vi "USBCom.vi"(0 "VISA resource name":refnum<visa-resource-name>, 5 "command":string, 11 "error in (no error)":errorcluster) -> (15 "error out":errorcluster)   [LabVIEW 2018]
uses:
  <vilib>/Instr/_visa.llb/VISA Flush IO Buffer Mask.ctl
  <vilib>/Instr/_visa.llb/VISA Configure Serial Port (Instr).vi
panel:
  in  "Add 0D0A":bool
  out "write buffer":string
  out "binary[7]":string
  out "number[7]":u32
  out "byte[7]":string
  out "number[4]":u32
  out "number[5]":u32
  out "number[6]":u32
  out "binary[6]":string
  out "byte[6]":string
  out "binary[5]":string
  out "byte[5]":string
  out "byte[4]":string
  out "binary[4]":string
  in  "resetValues":bool
  out "binary[3]":string
  out "number[3]":u32
  out "byte[3]":string
  out "number[0]":u32
  out "number[1]":u32
  out "number[2]":u32
  out "binary[2]":string
  out "byte[2]":string
  out "binary[1]":string
  out "byte[1]":string
  out "byte[0]":string
  out "binary[0]":string
  out "byte Array":string[](array[string])
  out "valid byte":string
  out "bytes at port":u32
  out "byte count":u32
  out "read buffer":string
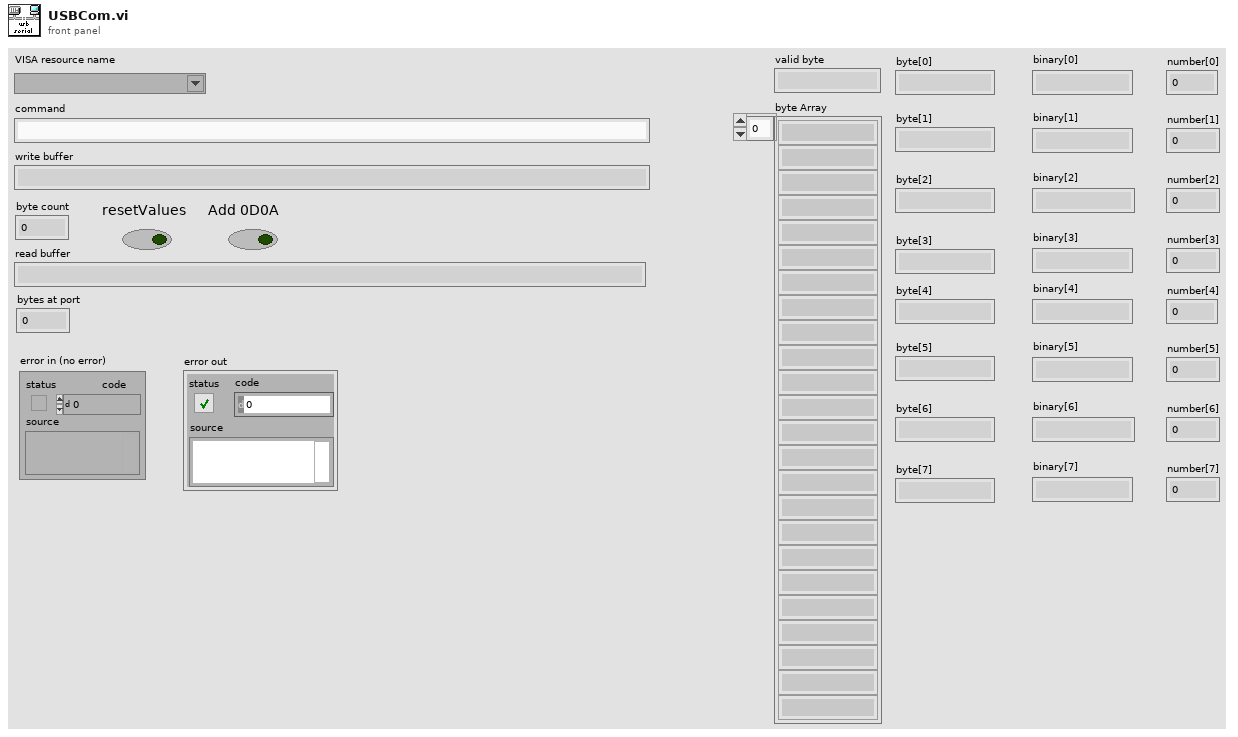
[diagram p1: front panel]
types:
  T1 = typedef "VISA Flush IO Buffer Mask.ctl" = u16
  T2 = cluster{"[0]":string, "[1]":string, "[2]":string, "[3]":string, "[4]":string, "[5]":string, "[6]":string, "[7]":string, "[8]":string}
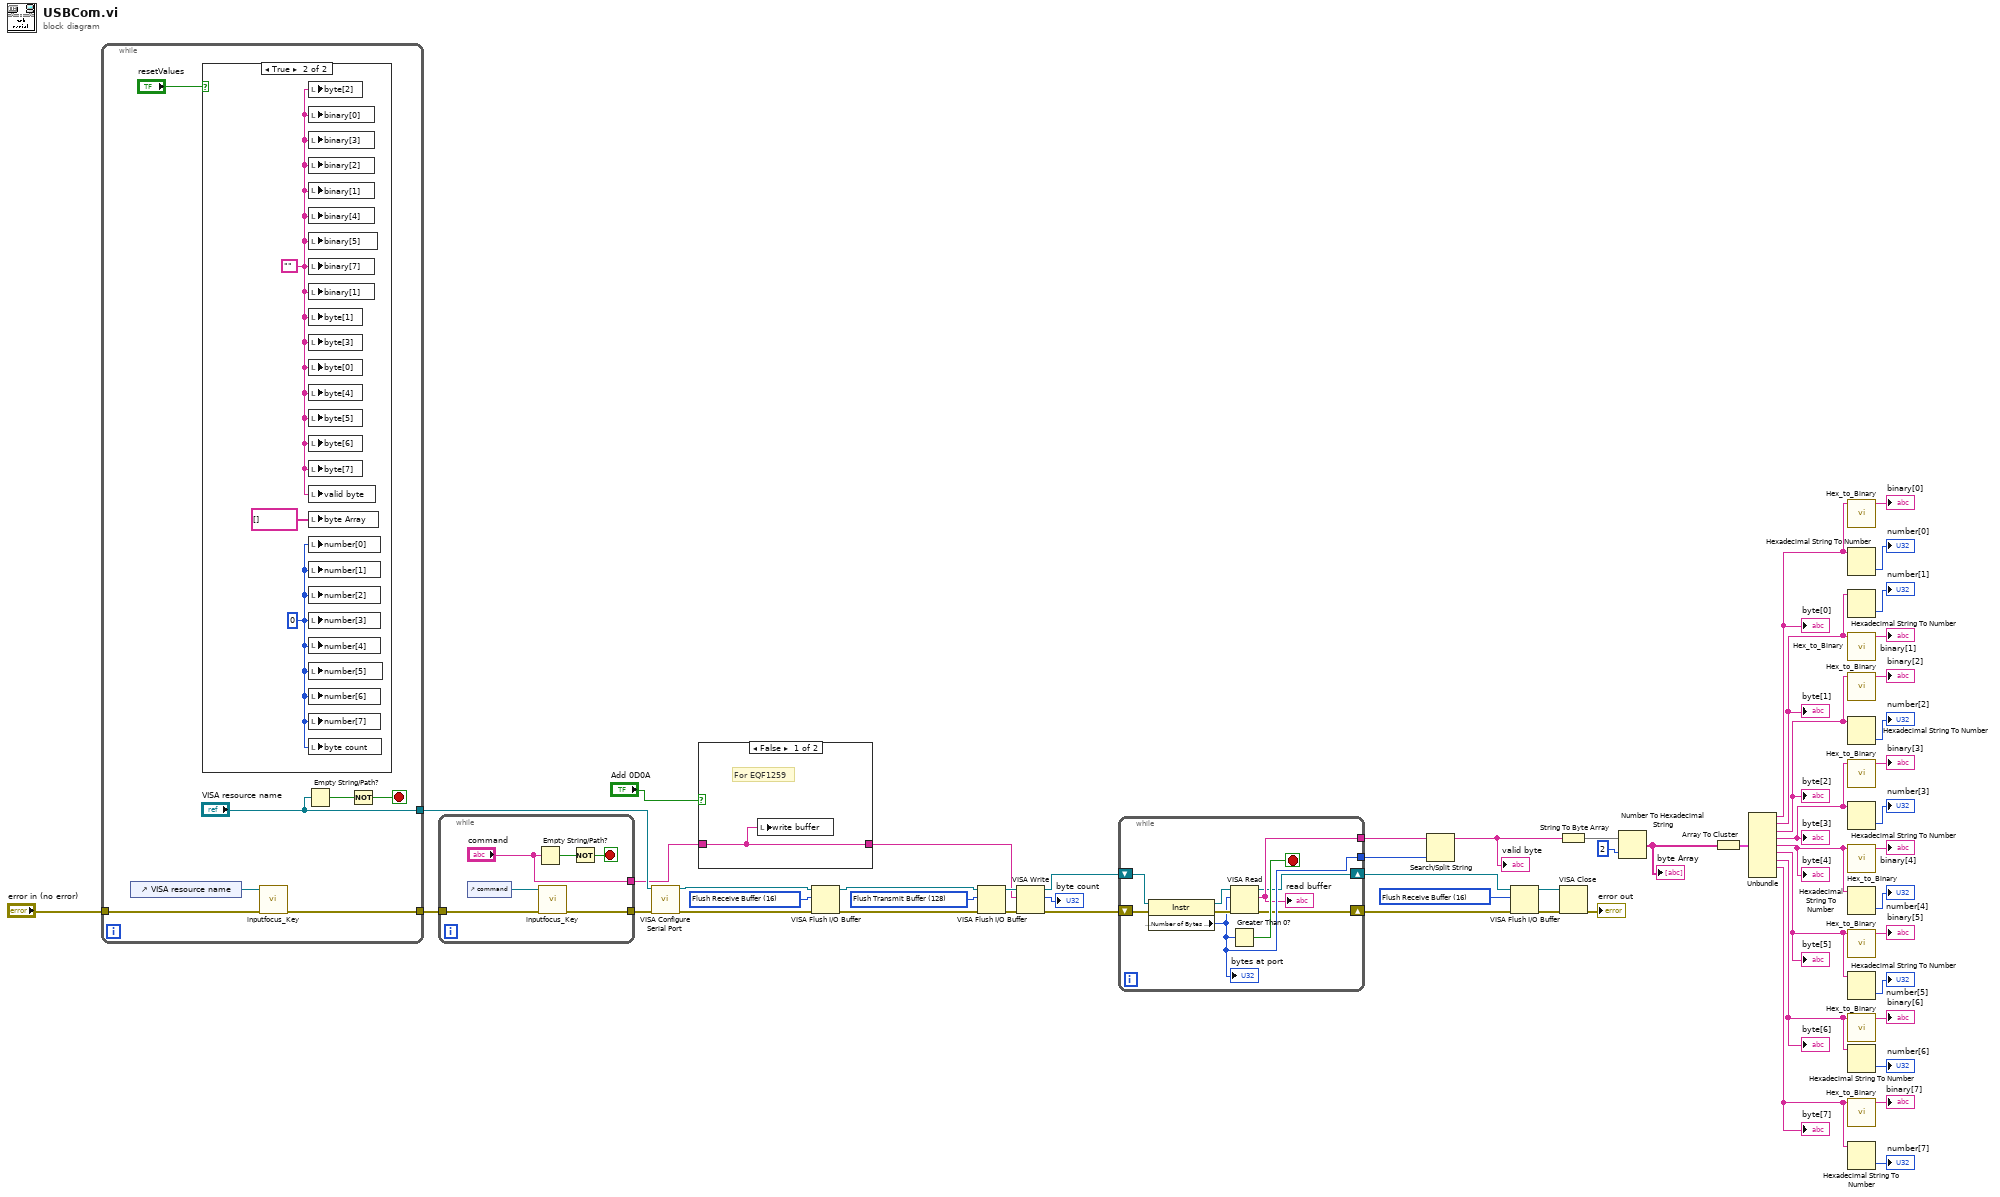
[diagram p0: block diagram]
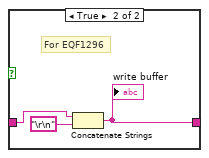
[diagram p2: hidden frame]
diagram:
  w39 = T1 128 items=["Flush Receive Buffer"=16, "Write Transmit Buffer to Device"=32, "Flush Receive Buffer (No I/O)"=64, "Flush Transmit Buffer"=128] ("Mask")
  w43 = T1 16 items=["Flush Receive Buffer"=16, "Write Transmit Buffer to Device"=32, "Flush Receive Buffer (No I/O)"=64, "Flush Transmit Buffer"=128] ("Mask")
  w46 = T1 16 items=["Flush Receive Buffer"=16, "Write Transmit Buffer to Device"=32, "Flush Receive Buffer (No I/O)"=64, "Flush Transmit Buffer"=128] ("Mask")
  n1 = while {
    tunnel: ["VISA resource name"] -> w33
    tunnel: [w62] -> w32
    tunnel: "error in (no error)" -> [w61]
    stop <- w57 stop-if-true
    n2 = control-ref of="VISA resource name"() -> (w60:refnum<vi>)
    n3 = case shown="True" "resetValues" {
      frame False {
      }
      frame True {
        w64 = u32 0
        w63 = ""
        n4 = local write "byte[2]"(w63) -> ()
        n5 = local write "binary[0]"(w63) -> ()
        n6 = local write "binary[3]"(w63) -> ()
        n7 = local write "binary[2]"(w63) -> ()
        n8 = local write "binary[1]"(w63) -> ()
        n9 = local write "binary[4]"(w63) -> ()
        n10 = local write "binary[5]"(w63) -> ()
        n11 = local write "binary[7]"(w63) -> ()
        n12 = local write "binary[1]"(w63) -> ()
        n13 = local write "byte[1]"(w63) -> ()
        n14 = local write "byte[3]"(w63) -> ()
        n15 = local write "byte[0]"(w63) -> ()
        n16 = local write "byte[4]"(w63) -> ()
        n17 = local write "byte[5]"(w63) -> ()
        n18 = local write "byte[6]"(w63) -> ()
        n19 = local write "byte[7]"(w63) -> ()
        n20 = local write "valid byte"(w63) -> ()
        n21 = local write "byte Array"(string[] []) -> ()
        n22 = local write "number[0]"(w64) -> ()
        n23 = local write "number[1]"(w64) -> ()
        n24 = local write "number[2]"(w64) -> ()
        n25 = local write "number[3]"(w64) -> ()
        n26 = local write "number[4]"(w64) -> ()
        n27 = local write "number[5]"(w64) -> ()
        n28 = local write "number[6]"(w64) -> ()
        n29 = local write "number[7]"(w64) -> ()
        n30 = local write "byte count"(w64) -> ()
      }
    }
    n31 = call "inputfocus_Key.vi"("error in (no error)"=w61, "reference"=w60) -> ("error out"=w62:errorcluster)  [unwired: 9 in]
    n32 = Empty String/Path?(string/path="VISA resource name") -> (empty?=w58:bool)
    n33 = Not(x=w58) -> (.not. x?=w57:bool)
  }
  n34 = while {
    tunnel: ["command"] -> w3
    tunnel: w32 -> [w71]
    tunnel: [w70] -> w31
    stop <- w66 stop-if-true
    n35 = control-ref of="command"() -> (w69:refnum<vi>)
    n36 = Empty String/Path?(string/path="command") -> (empty?=w67:bool)
    n37 = call "inputfocus_Key.vi"("error in (no error)"=w71, "reference"=w69) -> ("error out"=w70:errorcluster)  [unwired: 9 in]
    n38 = Not(x=w67) -> (.not. x?=w66:bool)
  }
  n39 = call-poly "VISA Configure Serial Port"("VISA resource name"=w33, "error in (no error)"=w31) -> ("VISA resource name out"=w45:refnum<visa-resource-name>, "error out"=w44:errorcluster)  [unwired: 12 in]
  n40 = case shown="False" "Add 0D0A" {
    tunnel: w3 -> [w72 w74]
    tunnel: [w72 w73] -> w2
    frame False {
      # "For EQF1259"
      n41 = local write "write buffer"(w72) -> ()
    }
    frame True {
      # "For EQF1296"
      n42 = Concatenate Strings(w74, "\r\n") -> (w73:string)
      "write buffer" <- w73
    }
  }
  n43 = VISA Flush I/O Buffer(VISA resource name=w45, mask (16)=w43, error in (no error)=w44) -> (VISA resource name out=w40:refnum<visa-resource-name>, error out=w41:errorcluster)
  n44 = VISA Flush I/O Buffer(VISA resource name=w40, mask (16)=w39, error in (no error)=w41) -> (VISA resource name out=w38:refnum<visa-resource-name>, error out=w37:errorcluster)
  n45 = VISA Write(VISA resource name=w38, write buffer=w2, error in (no error)=w37) -> (VISA resource name out=w55:refnum<visa-resource-name>, return count=→"byte count":u32, error out=w54:errorcluster)
  n46 = while {
    tunnel: [w78] -> w4
    tunnel: [w79] -> w50
    shift-right: [w76] -> w42
    shift-left: w55 -> [w84]
    shift-right: [w77] -> w47
    shift-left: w54 -> [w83]
    stop <- w80 stop-if-true
    n47 = property class="Instr"(reference=w84, error in=w83) -> (reference out=w81:refnum<visa-resource-name>, error out=w82:errorcluster, "Serial Settings:Number of Bytes at Serial Port"=w79:u32)
    "bytes at port" <- w79
    n48 = Greater Than 0?(x=w79) -> (x > 0?=w80:bool)
    n49 = VISA Read(VISA resource name=w81, byte count=w79, error in (no error)=w82) -> (VISA resource name out=w76:refnum<visa-resource-name>, read buffer=w78:string, error out=w77:errorcluster)  [unwired: 1 out]
    "read buffer" <- w78
  }
  n50 = Search/Split String(string=w4, offset (0)=w50) -> (substring before match=w48:string)  [unwired: 1 in, 2 out]
  "valid byte" <- w48
  n51 = VISA Flush I/O Buffer(VISA resource name=w42, mask (16)=w46, error in (no error)=w47) -> (VISA resource name out=w36:refnum<visa-resource-name>, error out=w35:errorcluster)
  n52 = String To Byte Array(string=w48) -> (unsigned byte array=w52:u8[])
  n53 = VISA Close(VISA resource name=w36, error in (no error)=w35) -> (error out=→"error out":errorcluster)
  n54 = Number To Hexadecimal String(1:i16 2 ("width (-)"), 2:w52) -> (0:w51:string[])
  "byte Array" <- w51
  n55 = Array To Cluster(array=w51) -> (cluster=w19:T2)
  n56 = Unbundle(w19) -> ("[0]"=w20:string, "[1]"=w21:string, "[2]"=w27:string, "[3]"=w17:string, "[4]"=w12:string, "[5]"=w11:string, "[6]"=w10:string, "[7]"=w9:string)  [unwired: 1 out]
  "byte[0]" <- w20
  "byte[1]" <- w21
  "byte[2]" <- w27
  "byte[3]" <- w17
  "byte[4]" <- w12
  "byte[5]" <- w11
  "byte[6]" <- w10
  "byte[7]" <- w9
  n57 = call "Hex_to_Binary.vi"("Hexadecimal String"=w20) -> ("Binary String"=→"binary[0]":string)  [unwired: 6 in, 2 out]
  n58 = Hexadecimal String To Number(string=w20) -> (number=→"number[0]":u32)  [unwired: 2 in, 1 out]
  n59 = Hexadecimal String To Number(string=w21) -> (number=→"number[1]":u32)  [unwired: 2 in, 1 out]
  n60 = call "Hex_to_Binary.vi"("Hexadecimal String"=w21) -> ("Binary String"=→"binary[1]":string)  [unwired: 6 in, 2 out]
  n61 = call "Hex_to_Binary.vi"("Hexadecimal String"=w27) -> ("Binary String"=→"binary[2]":string)  [unwired: 6 in, 2 out]
  n62 = Hexadecimal String To Number(string=w27) -> (number=→"number[2]":u32)  [unwired: 2 in, 1 out]
  n63 = call "Hex_to_Binary.vi"("Hexadecimal String"=w17) -> ("Binary String"=→"binary[3]":string)  [unwired: 6 in, 2 out]
  n64 = Hexadecimal String To Number(string=w17) -> (number=→"number[3]":u32)  [unwired: 2 in, 1 out]
  n65 = call "Hex_to_Binary.vi"("Hexadecimal String"=w12) -> ("Binary String"=→"binary[4]":string)  [unwired: 6 in, 2 out]
  n66 = Hexadecimal String To Number(string=w12) -> (number=→"number[4]":u32)  [unwired: 2 in, 1 out]
  n67 = call "Hex_to_Binary.vi"("Hexadecimal String"=w11) -> ("Binary String"=→"binary[5]":string)  [unwired: 6 in, 2 out]
  n68 = Hexadecimal String To Number(string=w11) -> (number=→"number[5]":u32)  [unwired: 2 in, 1 out]
  n69 = call "Hex_to_Binary.vi"("Hexadecimal String"=w10) -> ("Binary String"=→"binary[6]":string)  [unwired: 6 in, 2 out]
  n70 = Hexadecimal String To Number(string=w10) -> (number=→"number[6]":u32)  [unwired: 2 in, 1 out]
  n71 = call "Hex_to_Binary.vi"("Hexadecimal String"=w9) -> ("Binary String"=→"binary[7]":string)  [unwired: 6 in, 2 out]
  n72 = Hexadecimal String To Number(string=w9) -> (number=→"number[7]":u32)  [unwired: 2 in, 1 out]
